vi "GE 5565PIORC.DMA.Read.vi"(8 "error in (no error)":errorcluster, 9 "timeout ms (1000)":u32=1000, 10 "DMA Transfer Spec":T1 {"Block Descriptors"."descriptor params"."data ptr (lower)" format="%.0x"; "Block Descriptors"."descriptor params"."data ptr (upper)" format="%.0x"; "Block Descriptors"."descriptor params"."data size" format="%.0x"; "Block Descriptors"."descriptor params"."next descriptor ptr" format="%.0x"; "Block Descriptors"."descriptor size" format="%08x"; "Block Descriptors"."descriptor ptr (RFM)" format="%08x"; "Block Descriptors"."descriptor ptr (VISA)" format="%08x"; "RFM offset" format="%08x"}, 11 "GE 5565PIORC in":refnum<class "GE 5565PIORC.lvclass">) -> (0 "error out":errorcluster, 1 "timed out?":bool, 2 "DMA Transfer Spec dup":T1 {"Block Descriptors"."descriptor params"."data ptr (lower)" format="%.0x"; "Block Descriptors"."descriptor params"."data ptr (upper)" format="%.0x"; "Block Descriptors"."descriptor params"."data size" format="%.0x"; "Block Descriptors"."descriptor params"."next descriptor ptr" format="%.0x"; "Block Descriptors"."descriptor size" format="%08x"; "Block Descriptors"."descriptor ptr (RFM)" format="%08x"; "Block Descriptors"."descriptor ptr (VISA)" format="%08x"; "RFM offset" format="%08x"}, 3 "GE 5565PIORC out":refnum<class "GE 5565PIORC.lvclass">)   [LabVIEW 2016, in "GE 5565PIORC.lvclass"]
doc: "Configures an RFM to Host DMA transfer as defined by <B>DMA Transfer Spec</B>, starts the transfer, and then waits for the transfer to complete."
uses:
  GE 5565PIORC.lvclass
  Typedefs/GE 5565PIORC.Typedef.DMA Transfer Spec.ctl
  Typedefs/GE 5565PIORC.Typedef.DMA Block Descriptor.ctl
  Typedefs/GE 5565PIORC.Typedef.DMA Block Descriptor Params.ctl
  GE 5565PIORC.lvclass/GE 5565PIORC.ctl
  Properties/Registers/GE 5565PIORC.Registers.DMADPR0.Direction of Transfer.Set.vi
  Properties/Registers/GE 5565PIORC.Registers.DMASIZ0.DMA Transfer Size.Set.vi
  GE 5565PIORC.DMA.Size.vi
  Properties/Registers/GE 5565PIORC.Registers.DMALADR0.Local Address Register.Set.vi
  Properties/Registers/GE 5565PIORC.Registers.DMAMODE0.Scatter-Gather Mode.Set.vi
  Properties/Registers/GE 5565PIORC.Registers.DMAPADR0.PCI Address Register.Set.vi
  GE 5565PIORC.DMA.Scatter-Gather.Link Block Descriptors.vi
  GE 5565PIORC.DMA.Scatter-Gather.Commit Linked Block Descriptors.vi
  Properties/Registers/GE 5565PIORC.Registers.DMADPR0.Channel 0 First Descriptor Address.Set.vi
  <vilib>/Utility/error.llb/Clear Errors.vi
  Properties/Registers/GE 5565PIORC.Registers.DMACSR0.Channel 0 Start.Set.vi
  GE 5565PIORC.Interrupts.Wait for Event.vi
  Properties/Registers/GE 5565PIORC.Registers.DMACSR0.Channel 0 Clear Interrupt.Set.vi
  Properties/Registers/GE 5565PIORC.Registers.Local Configuration.Read.vi
  Properties/Registers/GE 5565PIORC.Registers.Local Configuration.Read (U32).vi
  Properties/Registers/GE 5565PIORC.Registers.Local Configuration.Write.vi
  Properties/Registers/GE 5565PIORC.Registers.Local Configuration.Write (U32).vi
  GE 5565PIORC.Bit Manipulation.Set Bit.vi
  GE 5565PIORC.Bit Manipulation.Set Bit (U32).vi
  GE 5565PIORC.DMA.Scatter-Gather.Set Descriptor Params.vi
  Properties/Registers/GE 5565PIORC.Registers.Local Configuration.Read (U8).vi
  Properties/Registers/GE 5565PIORC.Registers.Local Configuration.Write (U8).vi
  GE 5565PIORC.Bit Manipulation.Set Bit (U8).vi
  GE 5565PIORC.Registers.Read.vi
  GE 5565PIORC.Registers.Read (U32).vi
  GE 5565PIORC.Registers.Write.vi
  GE 5565PIORC.Registers.Write (U32).vi
  GE 5565PIORC.Registers.Read (U8).vi
  GE 5565PIORC.Registers.Write (U8).vi
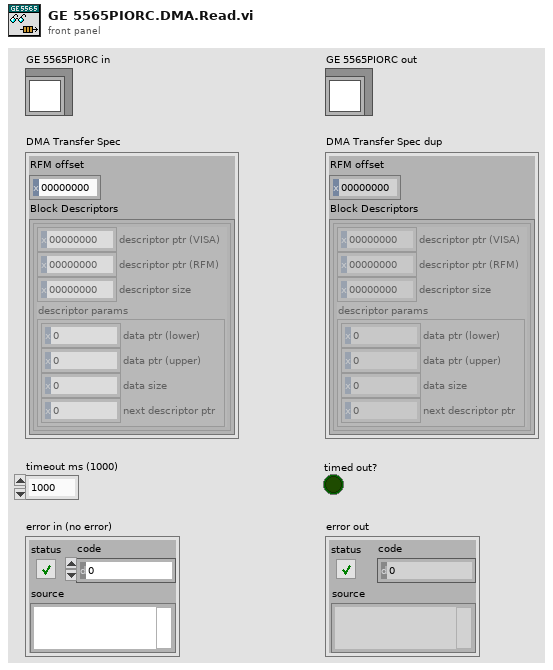
[diagram p1: front panel]
types:
  T1 = typedef "GE 5565PIORC.lvclass/GE 5565PIORC.Typedef.DMA Transfer Spec.ctl" = cluster{"RFM offset":u32, "Block Descriptors":T2[]}
  T2 = typedef "GE 5565PIORC.lvclass/GE 5565PIORC.Typedef.DMA Block Descriptor.ctl" = cluster{"descriptor ptr (VISA)":u32, "descriptor ptr (RFM)":u32, "descriptor size":u32, "descriptor params":T3}
  T3 = typedef "GE 5565PIORC.lvclass/GE 5565PIORC.Typedef.DMA Block Descriptor Params.ctl" = cluster{"data ptr (lower)":u32, "data ptr (upper)":u32, "data size":u32, "next descriptor ptr":u32}
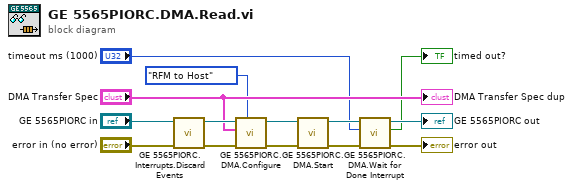
[diagram p0: block diagram]
diagram:
  n1 = call "GE 5565PIORC.Interrupts.Discard Events.vi"("error in (no error)"="error in (no error)", "GE 5565PIORC in"="GE 5565PIORC in") -> ("error out"=w11:errorcluster, "GE 5565PIORC out"=w12:refnum<class "GE 5565PIORC.lvclass">)  [unwired: 8 in]
  n2 = call "GE 5565PIORC.DMA.Configure.vi"("Transfer Direction"=enum16{"Host to RFM", "RFM to Host"}."RFM to Host", "error in (no error)"=w11, "DMA Transfer Spec"="DMA Transfer Spec", "GE 5565PIORC in"=w12) -> ("error out"=w10:errorcluster, "GE 5565PIORC out"=w9:refnum<class "GE 5565PIORC.lvclass">)  [unwired: 6 in]
  n3 = call "GE 5565PIORC.DMA.Start.vi"("error in (no error)"=w10, "GE 5565PIORC in"=w9) -> ("error out"=w7:errorcluster, "GE 5565PIORC out"=w8:refnum<class "GE 5565PIORC.lvclass">)  [unwired: 8 in]
  n4 = call "GE 5565PIORC.DMA.Wait for Done Interrupt.vi"("error in (no error)"=w7, "timeout ms (1000)"="timeout ms (1000)", "GE 5565PIORC in"=w8) -> ("error out"=→"error out":errorcluster, "timed out?"=→"timed out?":bool, "GE 5565PIORC out"=→"GE 5565PIORC out":refnum<class "GE 5565PIORC.lvclass">)  [unwired: 6 in]
  "DMA Transfer Spec dup" <- "DMA Transfer Spec"
